vi "Run Tests.vi"() -> ()   [LabVIEW 2019]
panel:
  out "Passed?":bool[](array[boolean])
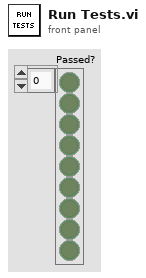
[diagram p1: front panel]
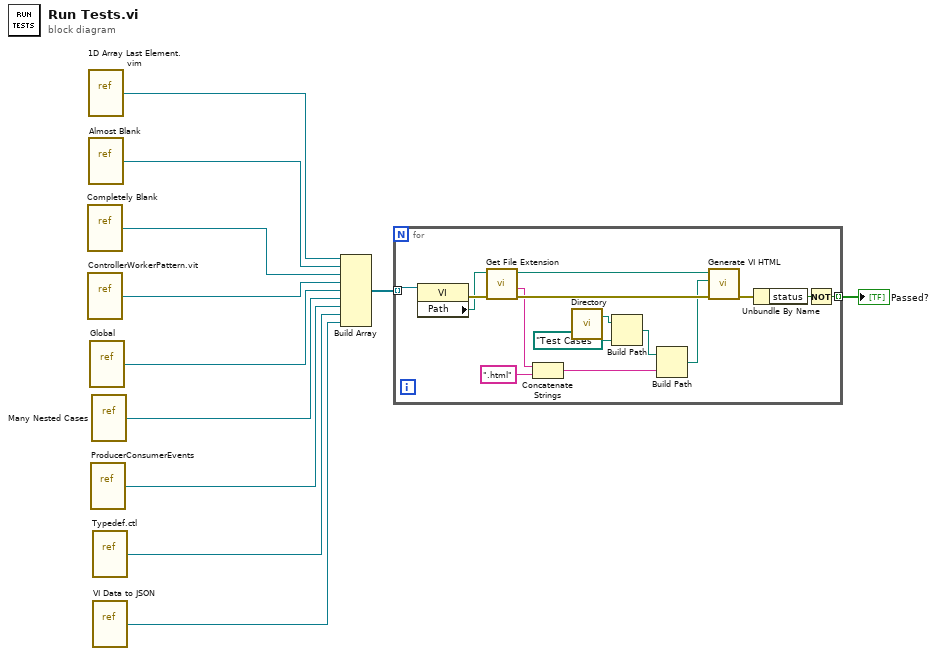
[diagram p0: block diagram]
diagram:
  n1 = vi-ref "Completely Blank.vi"() -> (w10:refnum<vi>)
  n2 = vi-ref "ControllerWorkerPattern.vit"() -> (w9:refnum<vi>)
  n3 = vi-ref "1D Array Last Element.vim"() -> (w2:refnum<vi>)
  n4 = vi-ref "Almost Blank.vi"() -> (w11:refnum<vi>)
  n5 = vi-ref "Global.vi"() -> (w8:refnum<vi>)
  n6 = vi-ref "ProducerConsumerEvents.vi"() -> (w7:refnum<vi>)
  n7 = vi-ref "Many Nested Cases.vi"() -> (w3:refnum<vi>)
  n8 = vi-ref "Typedef.ctl"() -> (w4:refnum<vi>)
  n9 = vi-ref "VI Data to JSON.vi"() -> (w1:refnum<vi>)
  n10 = Build Array(w2, w11, w10, w9, w8, w3, w7, w4, w1) -> (w6:refnum<vi>[])
  n11 = for {
    tunnel: w6 -> [w26] mode=indexing
    tunnel: [w16] -> w5 mode=indexing
    n12 = property class="VI"(reference=w26) -> (error out=w25:errorcluster, "Path"=w22:path)  [unwired: 1 in, 1 out]
    n13 = call <vilib>:"Get File Extension.vi"("error in (no error)"=w25, "file"=w22) -> ("error out"=w24:errorcluster, "filename without extension"=w21:string, "dup file"=w23:path)  [unwired: 5 in, 2 out]
    n14 = Concatenate Strings(w21, ".html" ("string")) -> (w19:string)
    n15 = call "Directory.vi"() -> ("Directory"=w14:path)  [unwired: 3 in]
    n16 = Build Path(base path=w14, name or relative path=path "Test Cases") -> (appended path=w12:path)
    n17 = Build Path(base path=w12, name or relative path=w19) -> (appended path=w18:path)
    n18 = call "Generate VI HTML.vi"("error in"=w24, "Output path"=w18, "VI Path"=w23) -> ("error out"=w15:errorcluster)  [unwired: 7 in, 1 out]
    n19 = Unbundle By Name(w15) -> ("status"=w17:bool)
    n20 = Not(x=w17) -> (.not. x?=w16:bool)
  }
  "Passed?" <- w5
